vi "Write Serial Configs.vi"(8 "error in (no error)":errorcluster, 10 "Item Ref in":T2 format="%.0x", 11 "Refnum in":T1) -> (0 "error out":errorcluster, 2 "Item Ref out":T2 format="%.0x", 3 "Refnum out":T1)   [LabVIEW 2015, in "Modbus Master System Explorer.lvlib"]
uses:
  Modbus Master System Explorer.lvlib
  <vilib>/Utility/config.llb/Config Data RefNum.ctl
  <vilib>/NI Veristand/Custom Device API/Custom Device Item Ref.ctl
  <vilib>/Utility/config.llb/Write Key (String).vi
  <vilib>/Utility/config.llb/Write Key (U32).vi
  <vilib>/Utility/config.llb/NI_LVConfig.lvlib
  <vilib>/NI VeriStand/Custom Device API/Custom Device API.lvlib
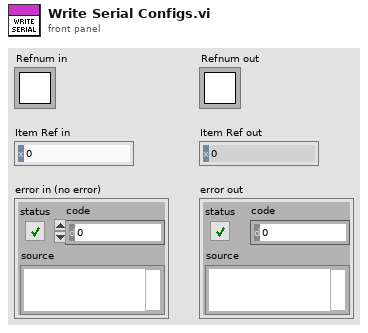
[diagram p1: front panel]
types:
  T1 = typedef "NI_LVConfig.lvlib/Config Data RefNum.ctl" = refnum<k1>
  T2 = typedef "Custom Device API.lvlib/Custom Device Item Ref.ctl" = u64
  T3 = typedef "Modbus Master Shared.lvlib/Parity.ctl" = u16
  T4 = typedef "Modbus Master Shared.lvlib/Serial Type.ctl" = enum16{"RTU", "ASCII"}
  T5 = typedef "Modbus Master Shared.lvlib/Flow Control.ctl" = u16
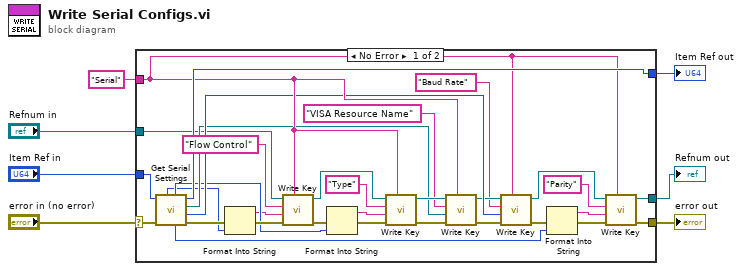
[diagram p0: block diagram]
diagram:
  n1 = case shown="No Error" "error in (no error)" {
    selector: "error in (no error)" -> [w9 w40]
    tunnel: [w39 w41] -> w7
    tunnel: [w37 w40] -> w6
    tunnel: [w36 w42] -> w5
    tunnel: "Serial" ("section") -> [w35 _]
    tunnel: "Item Ref in" -> [w10 w42]
    tunnel: "Refnum in" -> [w8 w41]
    frame No Error {
      n2 = call "Get Serial Settings.vi"("error in (no error)"=w9, "Item Ref in"=w10) -> ("error out"=w17:errorcluster, "baud rate"=w28:u32, "VISA resource name"=w22:refnum<visa-resource-name>, "Item Ref out"=w36:T2, "parity (even)"=w31:T3, "serial type"=w15:T4, "flow control (none)"=w12:T5)  [unwired: 3 in]
      n3 = Format Into String(error in=w17, w12) -> (resulting string=w13:string, error out=w18:errorcluster)  [unwired: 2 in]
      n4 = call-poly <vilib>:"Write Key.vi"("section"=w35, "error in (no error)"=w18, "value"=w13, "key"="Flow Control", "refnum"=w8) -> ("error out"=w19:errorcluster, "refnum out"=w25:T1)  [unwired: 4 in, 1 out]
      n5 = Format Into String(error in=w19, w15) -> (resulting string=w16:string, error out=w20:errorcluster)  [unwired: 2 in]
      n6 = call-poly <vilib>:"Write Key.vi"("section"=w35, "error in (no error)"=w20, "value"=w16, "key"="Type", "refnum"=w25) -> ("error out"=w23:errorcluster, "refnum out"=w24:T1)  [unwired: 4 in, 1 out]
      n7 = call-poly <vilib>:"Write Key.vi"("section"=w35, "error in (no error)"=w23, "value"=w22, "key"="VISA Resource Name", "refnum"=w24) -> ("error out"=w29:errorcluster, "refnum out"=w27:T1)  [unwired: 4 in, 1 out]
      n8 = call-poly <vilib>:"Write Key.vi"("section"=w35, "error in (no error)"=w29, "value"=w28, "key"="Baud Rate", "refnum"=w27) -> ("error out"=w33:errorcluster, "refnum out"=w38:T1)  [unwired: 4 in, 1 out]
      n9 = Format Into String(error in=w33, w31) -> (resulting string=w32:string, error out=w34:errorcluster)  [unwired: 2 in]
      n10 = call-poly <vilib>:"Write Key.vi"("section"=w35, "error in (no error)"=w34, "value"=w32, "key"="Parity", "refnum"=w38) -> ("error out"=w37:errorcluster, "refnum out"=w39:T1)  [unwired: 4 in, 1 out]
    }
    frame Error {
    }
  }
  "Refnum out" <- w7
  "error out" <- w6
  "Item Ref out" <- w5
